vi "Read Table Reference.vi"(11 "LookupTable in":refnum<class "LookupTable.lvclass">) -> (2 "Table Reference":refnum<data-value>, 3 "LookupTable out":refnum<class "LookupTable.lvclass">)   [LabVIEW 2020, in "LookupTable.lvlib" / "LookupTable.lvclass"]
uses:
  <vilib>/gpm_packages/@cs/lookup-table/Source/LookupTable/LookupTable.lvclass
  <vilib>/gpm_packages/@cs/lookup-table/Source/LookupTable/LookupTable.lvclass/LookupTable.ctl
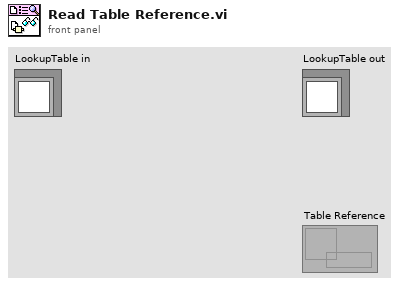
[diagram p1: front panel]
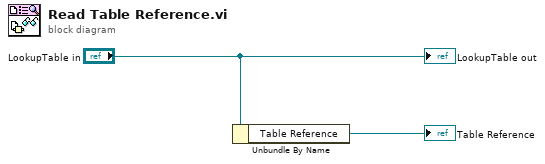
[diagram p0: block diagram]
diagram:
  n1 = Unbundle By Name("LookupTable in") -> ("Table Reference"=→"Table Reference":refnum<data-value>)
  "LookupTable out" <- "LookupTable in"
